vi "Error Query.vi"(8 "error in (no error)":errorcluster, 11 "VISA resource name":refnum<visa-resource-name>) -> (0 "error out":errorcluster, 1 "Error Message":string, 3 "VISA resource name out":refnum<visa-resource-name>)   [LabVIEW 2017, in "Stanford Research 830.lvlib"]
doc: "This VI queries the instrument for any errors in the instrument's error registers. It will continue to read errors until all errors have been read from the instrument. Any errors will be returned in the Error Out cluster.\n\n<B>Note:</B>\n\nThis VI is called automatically by most driver VIs so it is not usually necessary to call this in an application."
uses:
  Stanford Research 830.lvlib
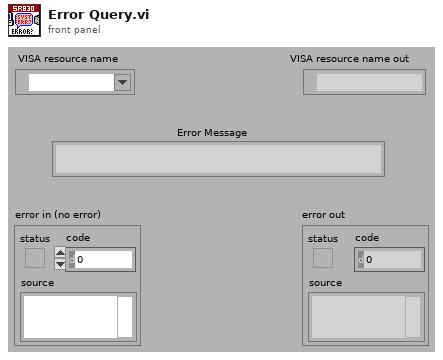
[diagram p1: front panel]
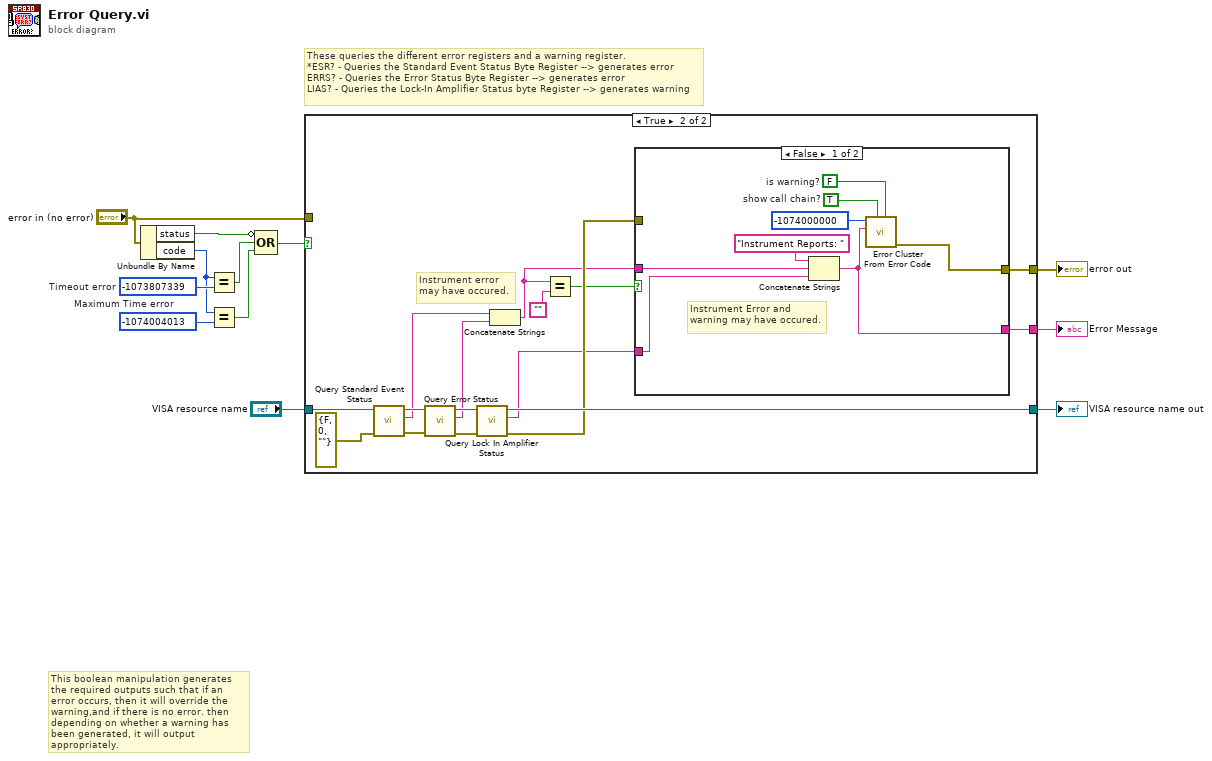
[diagram p0: block diagram]
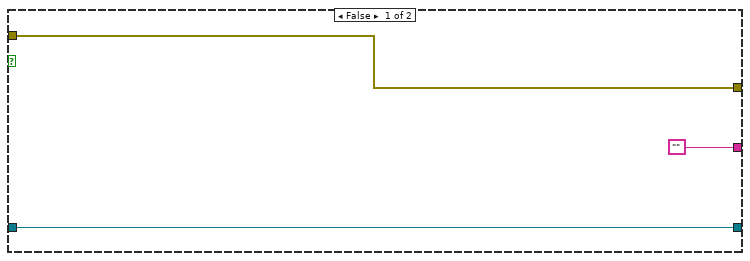
[diagram p2: hidden frame]
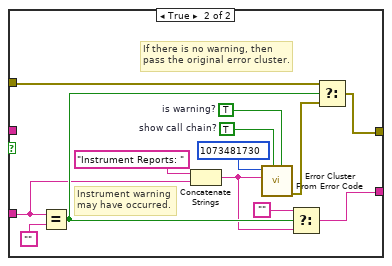
[diagram p3: hidden frame]
diagram:
  w3 = -1074004013  # Maximum Time error
  w11 = -1073807339  # Timeout error
  # "This boolean manipulation generates the required outputs such that if an error occurs, then it will override the warning,and if there is no error. then depending on whether a warning has been generated, it will output appropriately."
  # "These queries the different error registers and a warning register. \n*ESR? - Queries the Standard Event Status Byte Register --> generates error\nERRS? - Queries the Error Status Byte Register --> generates error\nLIAS? - Queries the Lock-In Amplifier Status byte Register --> generates warning"
  n1 = Unbundle By Name("error in (no error)") -> ("status"=w12:bool, "code"=w2:i32)
  n2 = Equal?(x=w2, y=w11) -> (x = y?=w10:bool)
  n3 = Equal?(x=w2, y=w3) -> (x = y?=w1:bool)
  n4 = Compound Arithmetic op=OR(invert w12, w10, w1) -> (w9:bool)
  n5 = case shown="True" w9 {
    tunnel: "VISA resource name" -> [w15 w31]
    tunnel: "error in (no error)" -> [w14 _]
    tunnel: ["" w24] -> w6
    tunnel: [w14 w26] -> w5
    tunnel: [w15 w27] -> w4
    frame False {
    }
    frame True {
      # "Instrument error may have occured."
      n6 = call "Query Standard Event Status.vi"("error in (no error)"=errorcluster {"status"=FALSE, "code"=0, "source"=""}, "VISA resource name"=w31) -> ("error out"=w23:errorcluster, "Standard Event Status Data Message"=w21:string, "VISA resource name out"=w30:refnum<visa-resource-name>)  [unwired: 7 in]
      n7 = call "Query Error Status.vi"("error in (no error)"=w23, "VISA resource name"=w30) -> ("error out"=w22:errorcluster, "Error Status Data Message"=w20:string, "VISA resource name out"=w28:refnum<visa-resource-name>)  [unwired: 7 in]
      n8 = call "Query Lock In Amplifier Status.vi"("error in (no error)"=w22, "VISA resource name"=w28) -> ("error out"=w25:errorcluster, "Lock In Amplifier Data Message"=w16:string, "VISA resource name out"=w27:refnum<visa-resource-name>)  [unwired: 7 in]
      n9 = Concatenate Strings(w21, w20) -> (w17:string)
      n10 = Equal?(x=w17, y="") -> (x = y?=w18:bool)
      n11 = case shown="False" w18 {
        tunnel: [w36 w49] -> w26
        tunnel: w25 -> [_ w40]
        tunnel: [w35 w48] -> w24
        tunnel: w17 -> [w33 _]
        tunnel: w16 -> [w32 w44]
        frame False {
          w37 = FALSE  # is warning?
          w38 = TRUE  # show call chain?
          # "Instrument Error and warning may have occured."
          n12 = Concatenate Strings("Instrument Reports: " ("string"), w33, w32) -> (w35:string)
          n13 = call <vilib>:"Error Cluster From Error Code.vi"("is warning? (False)"=w37, "show call chain? (False)"=w38, "error message (\"\")"=w35, "error code (0)"=-1074000000 ("t")) -> ("error out"=w36:errorcluster)  [unwired: 5 in]
        }
        frame True {
          w50 = TRUE  # is warning?
          w51 = TRUE  # show call chain?
          # "If there is no warning, then pass the original error cluster."
          # "Instrument warning may have occurred."
          n14 = Equal?(x=w44, y="") -> (x = y?=w45:bool)
          n15 = Concatenate Strings("Instrument Reports: " ("string"), w44) -> (w42:string)
          n16 = call <vilib>:"Error Cluster From Error Code.vi"("is warning? (False)"=w50, "show call chain? (False)"=w51, "error message (\"\")"=w42, "error code (0)"=1073481730 ("t")) -> ("error out"=w41:errorcluster)  [unwired: 5 in]
          n17 = Select(t="" ("f"), s=w45, f=w42) -> (s? t:f=w48:string)
          n18 = Select(t=w40, s=w45, f=w41) -> (s? t:f=w49:errorcluster)
        }
      }
    }
  }
  "error out" <- w5
  "VISA resource name out" <- w4
  "Error Message" <- w6
